vi "onCreated.vi"(8 "error in (no error)":errorcluster, 11 "system":refnum<class "system.lvclass">) -> (0 "error out":errorcluster, 3 "system out":refnum<class "system.lvclass">)   [LabVIEW 2020, in "system.lvclass"]
doc: "JKI State Machine Objects (SMO) 1.2.1.55\nJKI - JKI\nCopyright (c) 2017, JKI"
uses:
  system.lvclass
  DSP/DSP.lvclass
  C:/Program Files (x86)/National Instruments/LabVIEW 2020/vi.lib/JKI/JKI SMO/SMO/SMO.lvclass
  DAQ_Manager/DAQ_Manager.lvclass
  Generator/Generator.lvclass
  Scope/Scope.lvclass
  system.lvclass/system.ctl
  instrument/instrument.lvclass
  <vilib>/JKI/JKI SMO/SMO/SMO.lvclass
panel:
  # "For instructions on how to use the JKI State Machine Objects, examples and video tutorials, visit:\nhttp://jki.net/state-machine-objects/\n\nJKI State Machine Objects™\nhttp://jki.net/state-machine-objects/\nCopyright (C) 2005-2015, JKI <info@jki.net>\nALL RIGHTS RESERVED"
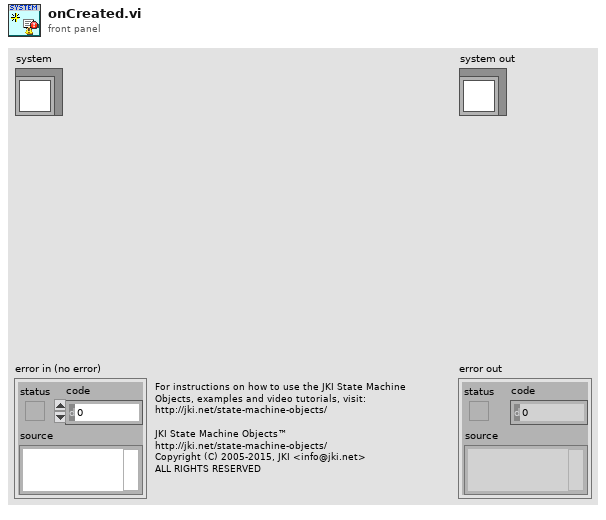
[diagram p1: front panel]
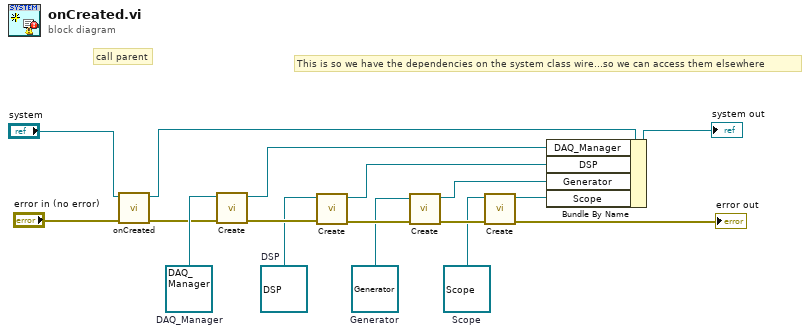
[diagram p0: block diagram]
diagram:
  w1 = refnum<class "Scope.lvclass"> refnum  # Scope
  w8 = refnum<class "Generator.lvclass"> refnum  # Generator
  w13 = refnum<class "DAQ_Manager.lvclass"> refnum  # DAQ_Manager
  w9 = refnum<class "DSP.lvclass"> refnum  # DSP
  # "call parent"
  # "This is so we have the dependencies on the system class wire...so we can access them elsewhere"
  n1 = call-parent "onCreated.vi"("error in (no error)"="error in (no error)", "SMO"="system") -> ("error out"=w12:errorcluster, "SMO out"=w15:refnum<class "system.lvclass">)  [unwired: 8 in]
  n2 = call <vilib>:"Create.vi"("error in (no error)"=w12, "SMO"=w13) -> ("error out"=w11:errorcluster, "SMO out"=w6:refnum<class "DAQ_Manager.lvclass">)  [unwired: 7 in, 1 out]
  n3 = call <vilib>:"Create.vi"("error in (no error)"=w11, "SMO"=w9) -> ("error out"=w10:errorcluster, "SMO out"=w7:refnum<class "DSP.lvclass">)  [unwired: 7 in, 1 out]
  n4 = call <vilib>:"Create.vi"("error in (no error)"=w10, "SMO"=w8) -> ("error out"=w4:errorcluster, "SMO out"=w5:refnum<class "Generator.lvclass">)  [unwired: 7 in, 1 out]
  n5 = call <vilib>:"Create.vi"("error in (no error)"=w4, "SMO"=w1) -> ("error out"=→"error out":errorcluster, "SMO out"=w2:refnum<class "Scope.lvclass">)  [unwired: 7 in, 1 out]
  n6 = Bundle By Name(cluster=w15, "DAQ_Manager"=w6, "DSP"=w7, "Generator"=w5, "Scope"=w2) -> (→"system out":refnum<class "system.lvclass">)
